vi "Read azElParameters.vi"(8 "error in (no error)":errorcluster, 11 "AzElTarget in":refnum<class "AzElTarget.lvclass">) -> (0 "error out":errorcluster, 2 "AzElParameters.lvclass":refnum<class "AzElParameters.lvclass">, 3 "AzElTarget out":refnum<class "AzElTarget.lvclass">)   [LabVIEW 2022 SP3, in "TCSDataDefinitions.lvlib" / "TCSCommand.lvlib" / "TargetConfiguration.lvlib" / "Target.lvlib" / "FixedTarget.lvlib" / "AzElTarget.lvclass"]
uses:
  AzElTarget.lvclass
  AzElParameters/AzElParameters.lvclass
  AzElTarget.lvclass/AzElTarget.ctl
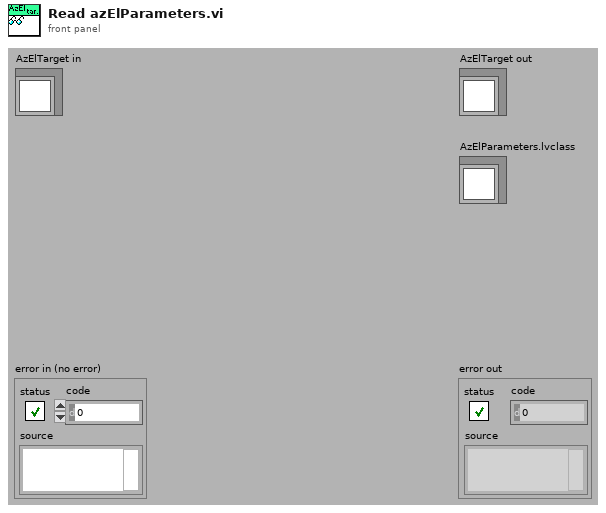
[diagram p1: front panel]
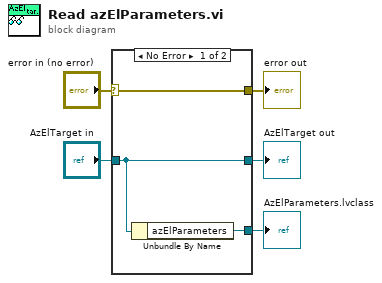
[diagram p0: block diagram]
diagram:
  n1 = case shown="No Error" "error in (no error)" {
    selector: "error in (no error)" -> [w8 w9]
    tunnel: [w8 w9] -> w4
    tunnel: [w7 w10] -> w2
    tunnel: "AzElTarget in" -> [w7 w10]
    tunnel: [w6 _] -> w1
    frame No Error {
      n2 = Unbundle By Name(w7) -> ("azElParameters"=w6:refnum<class "AzElParameters.lvclass">)
    }
    frame Error {
    }
  }
  "error out" <- w4
  "AzElTarget out" <- w2
  "AzElParameters.lvclass" <- w1
